vi "s-lab第7章 程序结构1-20.vi"() -> ()   [LabVIEW 2013]
uses:
  <vilib>/Platform/TimedLoop/XDataNode/timing_clust.ctl
  <vilib>/Platform/TimedLoop/XDataNode/nitl_modes.ctl
  <vilib>/Platform/TimedLoop/XDataNode/wakeup.ctl
  <vilib>/Platform/TimedLoop/XDataNode/XDataNode.xnode
  <vilib>/Platform/TimedLoop/XDataNode/XDNodeRunTimeDep.lvlib
panel:
  out "平方根":dbl
  in  "数值 8":dbl
  out "判断结果":dbl
  in  "比较门限":dbl
  out "随机数":dbl
  out "滑动杆值":dbl
  out "布尔 4":bool
  in  "数值 7":dbl
  in  "滑动杆 3":dbl(slide) scale=0.0..10.0
  out "字符串 5":string
  out "0-n的平方和":dbl
  in  "输入n":dbl
  out "0-99之间的所有偶数之和":dbl
  in  "循环值":dbl
  out "小数":dbl
  out "大数":dbl
  out "循环次数":dbl
  out "字符串 4":string
  in  "字符串 3":string
  out "数值 6":dbl
  in  "数值 5":dbl
  in  "确定按钮":bool
  in  "滑动杆 2":dbl(slide) scale=0.0..10.0
  out "OUT":dbl
  in  "IN":dbl
  out "延迟时间 S 2":dbl
  in  "数值 4":dbl
  out "延迟时间 S":dbl
  in  "数值 3":dbl
  out "数值 2":dbl
  out "字符串 2":string
  in  "停止 2":bool
  out "布尔":bool
  in  "数值":dbl
  in  "滑动杆":dbl(slide) scale=0.0..10.0
  in  "布尔 3":bool
  out "字符串":string
  out "布尔 2":bool
  out "n的和 1":dbl
  in  "数值n 2":dbl
  out "循环数2":dbl
  out "n！ 1":dbl
  in  "数值n 1":dbl
  in  "停止":bool
  out "随机数":dbl
  out "循环数":dbl
  out "n的和":dbl
  in  "数值n":dbl
  out "n！":dbl
  in  "n":dbl
  out "随机数":dbl
  out "循环":dbl
  # "例 1"
  # "例 2"
  # "例 3"
  # "例 4"
  # "例 5"
  # "例 6"
  # "例 7"
  # "例 8"
  # "例 9"
  # "例 10"
  # "例 11"
  # "例 12"
  # "例 13"
  # "例 14"
  # "例 15"
  # "例 16"
  # "例 17"
  # "例 18"
  # "例 19"
  # "例 20"
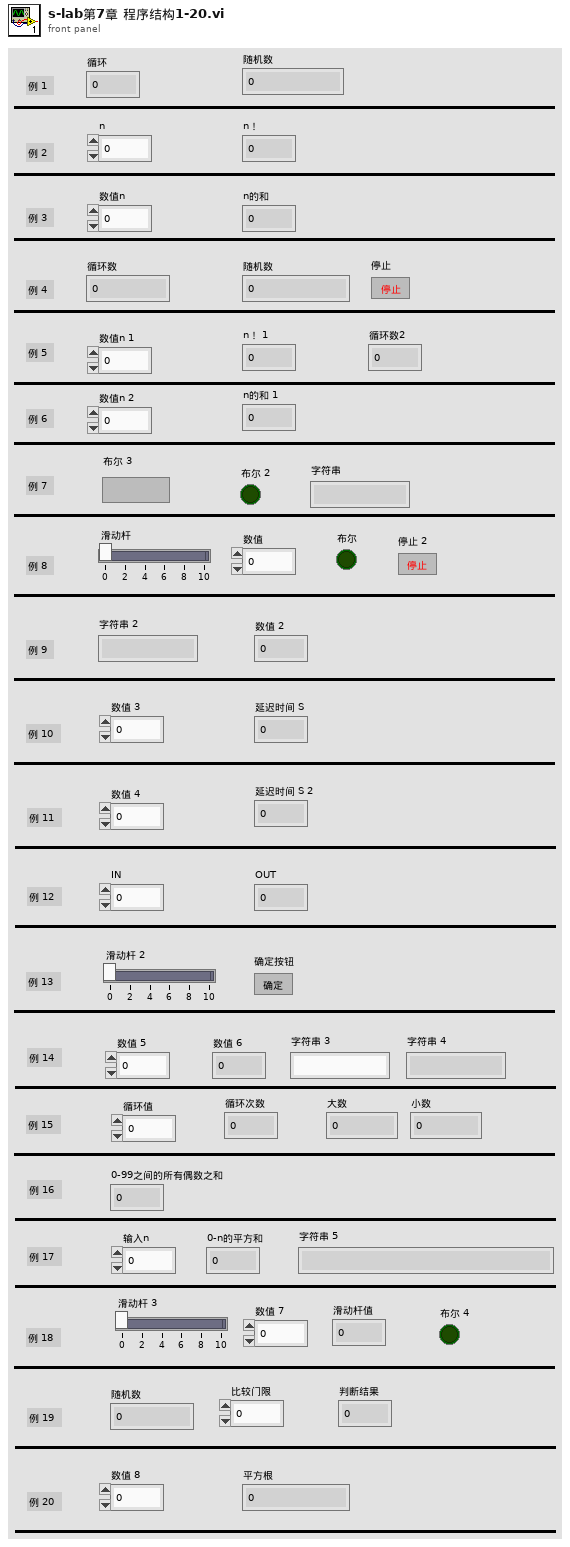
[diagram p1: front panel]
types:
  T1 = typedef "XDNodeRunTimeDep.lvlib/timing_clust.ctl" = cluster{"Expected End [f-1]":u64, "Actual End [f-1]":u64, "Finished Late? [f-1]":bool, "Expected End [i-1]":u64, "Actual End [i-1]":u64, "Finished Late? [i-1]":bool, "Expected Start [i]":u64, "Actual Start [i]":u64, "Expected Start [f]":u64, "Actual Start [f]":u64, "Source Name":string, "Structure Name":string, "Period":i64, "Deadline":i64, "Offset":i64, "Start":i64, "Priority":i32, "Timeout":i32, "Mode":T2, "Wakeup Reason":T3, "Error":errorcluster, "Source Type":string, "Secondary Source Type":string, "Global End Time":u64, "Global Start Time":u64, "Frame Duration":u64, "Iteration Duration":u64, "Assigned CPU":i32, "I/O Scan Engine Mode":u32}
  T2 = typedef "XDNodeRunTimeDep.lvlib/nitl_modes.ctl" = enum32{"No Change", "Process missed periods, maintain original phase", "Discard missed periods, maintain original phase", "Process missed periods, ignore original phase", "Discard missed periods, ignore original phase"}
  T3 = typedef "XDNodeRunTimeDep.lvlib/wakeup.ctl" = enum32{"Normal", "Aborted", "Asynchronous wakeup", "Timing source error", "Timed loop error", "Timeout"}
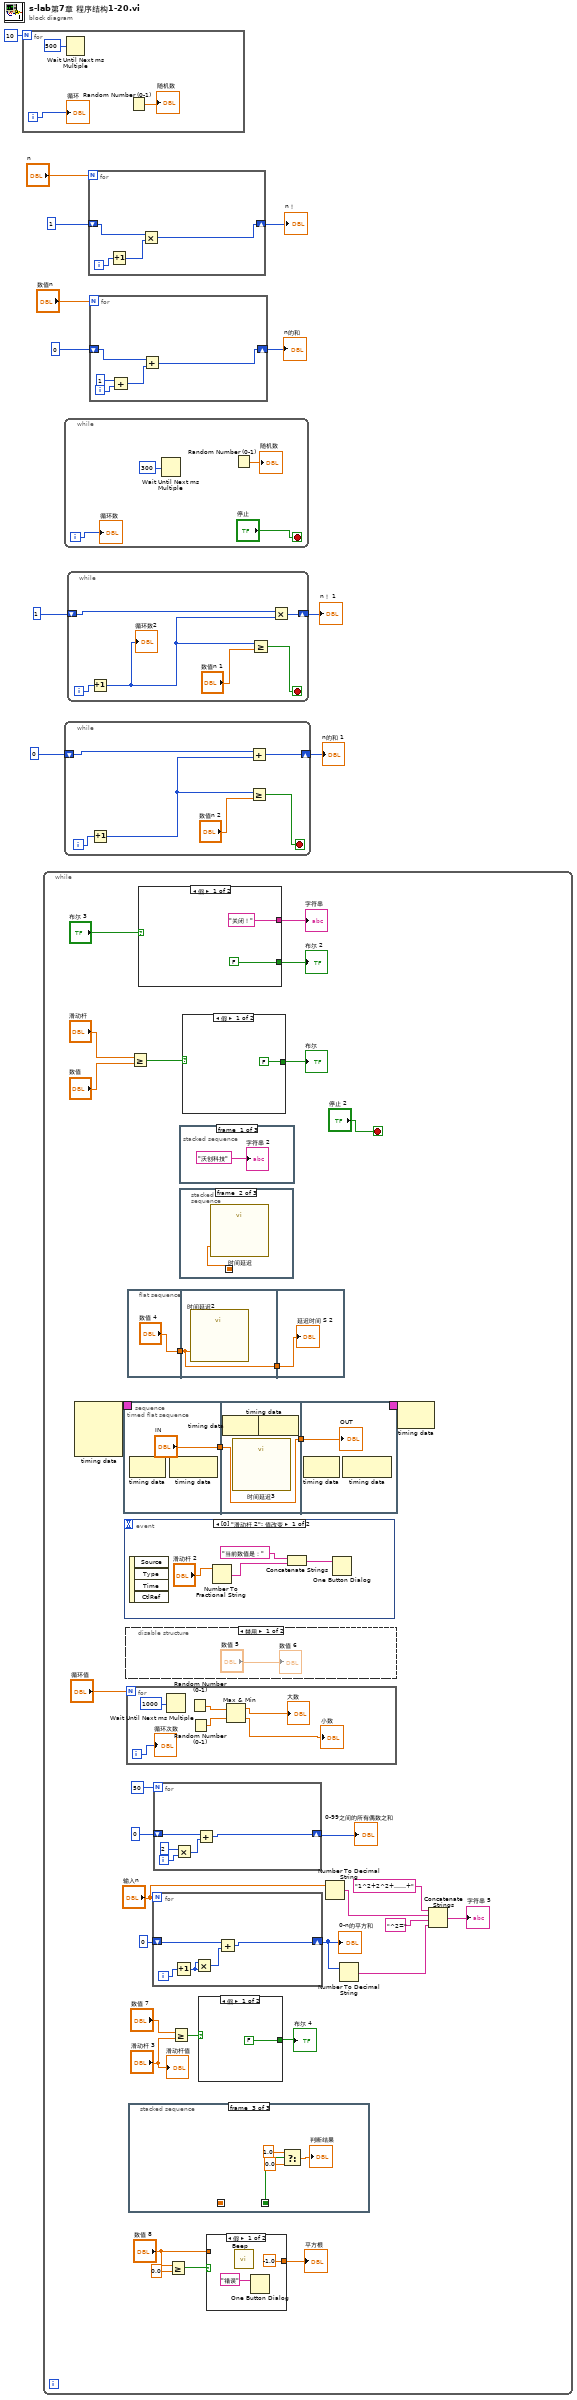
[diagram p0: block diagram]
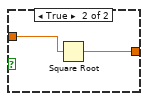
[diagram p2: hidden frame]
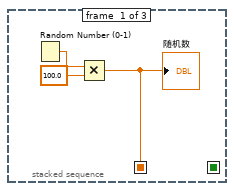
[diagram p3: hidden frame]
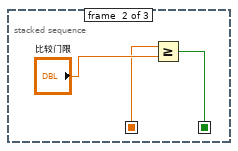
[diagram p4: hidden frame]
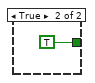
[diagram p5: hidden frame]
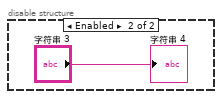
[diagram p6: hidden frame]
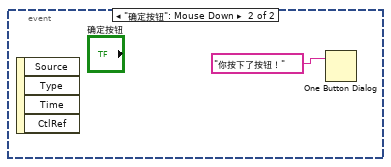
[diagram p7: hidden frame]
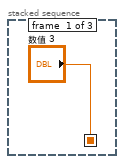
[diagram p8: hidden frame]
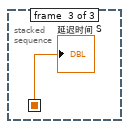
[diagram p9: hidden frame]
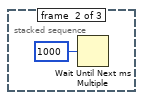
[diagram p10: hidden frame]
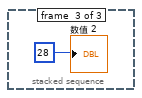
[diagram p11: hidden frame]
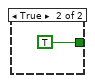
[diagram p12: hidden frame]
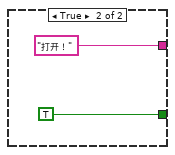
[diagram p13: hidden frame]
diagram:
  n1 = for {
    N: 10 -> [_]
    i -> [w12]
    n2 = Wait Until Next ms Multiple(millisecond multiple=u32 500 ("毫秒倍数")) -> ()  [unwired: 1 out]
    n3 = Random Number (0-1)() -> (number: 0 to 1=→"随机数":dbl)
    "循环" <- w12
  }
  n4 = while {
    stop <- "停止 2" stop-if-true
    n5 = node-c288() -> (w36:T1)  [unwired: 4 in]
    n6 = timed-sequence {
      timing: w36 -> [_]
      timing-out: [_] -> w35
      n7 = timed-flat-sequence {
        tunnel: ["IN"] -> w86
        tunnel: [w91] -> w87
        tunnel: w86 -> [w91]
        tunnel: w87 -> [w94]
        frame #0 {
          n8 = node-c288() -> ()  [unwired: 1 in, 1 out]
          n9 = node-c288() -> ()  [unwired: 1 in, 1 out]
        }
        frame #1 {
          n10 = node-c288() -> ()  [unwired: 1 in, 1 out]
          n11 = call "时间延迟3"() -> ()  [unwired: 11 in, 1 out]
          n12 = node-c288() -> ()  [unwired: 1 in, 1 out]
        }
        frame #2 {
          n13 = node-c288() -> ()  [unwired: 1 in, 1 out]
          n14 = node-c288() -> ()  [unwired: 1 in, 1 out]
          "OUT" <- w94
        }
      }
    }
    n15 = event shown="[0] \"滑动杆 2\": 值改变" {
      selector: _ -> [_ _]
      dyn-events: _ -> [_ _]
      timeout: _ -> [_ _]
      event "滑动杆 2": Value Change {
        n16 = event-data() -> ()  [unwired: 1 in, 4 out]
        n17 = Number To Fractional String(number="滑动杆 2") -> (F-format string=w83:string)  [unwired: 3 in]
        n18 = Concatenate Strings("当前数值是：", w83) -> (w81:string)
        n19 = One Button Dialog(message=w81) -> ()  [unwired: 1 in, 1 out]
      }
      event "确定按钮": Mouse Down {
        n20 = event-data() -> ()  [unwired: 1 in, 4 out]
        n21 = One Button Dialog(message="你按下了按钮！") -> ()  [unwired: 1 in, 1 out]
      }
    }
    n22 = disable-structure shown="禁用" {
      frame Disabled {
        "数值 6" <- "数值 5"
      }
      frame Enabled {
        "字符串 4" <- "字符串 3"
      }
    }
    n23 = for {
      N: "循环值" -> [_]
      i -> [w78]
      n24 = Wait Until Next ms Multiple(millisecond multiple=u32 1000 ("毫秒倍数")) -> ()  [unwired: 1 out]
      n25 = Random Number (0-1)() -> (number: 0 to 1=w77:dbl)
      n26 = Random Number (0-1)() -> (number: 0 to 1=w76:dbl)
      n27 = Max & Min(x=w77, y=w76) -> (max(x,y)=→"大数":dbl, min(x,y)=→"小数":dbl)
      "循环次数" <- w78
    }
    n28 = flat-sequence {
      tunnel: ["数值 4"] -> w38
      tunnel: w38 -> [w100]
      tunnel: [w100] -> w37
      tunnel: w37 -> [w101]
      frame #0 {
      }
      frame #1 {
        n29 = call "时间延迟2"("Delay Time (s)"=w100) -> ()  [unwired: 10 in, 1 out]
      }
      frame #2 {
        "延迟时间 S 2" <- w101
      }
    }
    n30 = stacked-sequence {
      seq-local: [w51 _ _] -> [_ w55 _]
      seq-local: [_ w54 _] -> [_ _ w59]
      frame #0 {
        n31 = Random Number (0-1)() -> (number: 0 to 1=w53:dbl)
        n32 = Multiply(x=w53, y=100.0) -> (x*y=w51:dbl)
        "随机数" <- w51
      }
      frame #1 {
        n33 = Greater Or Equal?(x=w55, y="比较门限") -> (x >= y?=w54:bool)
      }
      frame #2 {
        n34 = Select(t=1.0, s=w59, f=0.0) -> (s? t:f=→"判断结果":dbl)
      }
    }
    n35 = Greater Or Equal?(x="滑动杆", y="数值") -> (x >= y?=w43:bool)
    n36 = case shown="假" "布尔 3" {
      tunnel: [FALSE TRUE] -> w40
      tunnel: ["关闭！" "打开！"] -> w41
      frame False {
      }
      frame True {
      }
    }
    "布尔 2" <- w40
    "字符串" <- w41
    n37 = for {
      N: "输入n" -> [_]
      shift-right: [w63] -> w29
      shift-left: 0 -> [w64]
      i -> [w67]
      n38 = Increment(x=w67) -> (x+1=w66:i32)
      n39 = Multiply(x=w66, y=w66) -> (x*y=w65:i32)
      n40 = Add(x=w64, y=w65) -> (x+y=w63:i32)
    }
    "0-n的平方和" <- w29
    n41 = for {
      N: 50 -> [_]
      shift-right: [w68] -> w31
      shift-left: 0 -> [w69]
      i -> [w72]
      n42 = Multiply(x=2, y=w72) -> (x*y=w70:i32)
      n43 = Add(x=w69, y=w70) -> (x+y=w68:i32)
    }
    "0-99之间的所有偶数之和" <- w31
    n44 = Greater Or Equal?(x="数值 8", y=0.0) -> (x >= y?=w17:bool)
    n45 = Greater Or Equal?(x="数值 7", y="滑动杆 3") -> (x >= y?=w20:bool)
    n46 = stacked-sequence {
      seq-local: ["数值 3" _ _] -> [_ w103 w104]
      frame #0 {
      }
      frame #1 {
        n47 = call "时间延迟"("Delay Time (s)"=w103) -> ()  [unwired: 10 in, 1 out]
      }
      frame #2 {
        "延迟时间 S" <- w104
      }
    }
    n48 = stacked-sequence {
      frame #0 {
        "字符串 2" <- "沃创科技"
      }
      frame #1 {
        n49 = Wait Until Next ms Multiple(millisecond multiple=u32 1000 ("毫秒倍数")) -> ()  [unwired: 1 out]
      }
      frame #2 {
        "数值 2" <- 28
      }
    }
    n50 = case shown="假" w43 {
      tunnel: [FALSE TRUE] -> w46
      frame False {
      }
      frame True {
      }
    }
    "布尔" <- w46
    n51 = case shown="假" w20 {
      tunnel: [FALSE TRUE] -> w19
      frame False {
      }
      frame True {
      }
    }
    "布尔 4" <- w19
    n52 = case shown="假" w17 {
      tunnel: "数值 8" -> [_ w50]
      tunnel: [-1.0 w49] -> w15
      frame False {
        n53 = call <vilib>:"Beep.vi"() -> ()  [unwired: 12 in]
        n54 = One Button Dialog(message="错误") -> ()  [unwired: 1 in, 1 out]
      }
      frame True {
        n55 = Square Root(x=w50) -> (sqrt(x)=w49:dbl)
      }
    }
    "平方根" <- w15
    n56 = Number To Decimal String(number="输入n") -> (decimal integer string=w25:string)  [unwired: 1 in]
    n57 = Number To Decimal String(number=w29) -> (decimal integer string=w27:string)  [unwired: 1 in]
    n58 = node-c288(w35) -> ()  [unwired: 1 out]
    n59 = Concatenate Strings("1^2+2^2+……+", w25, "^2=", w27) -> (→"字符串 5":string)
    "滑动杆值" <- "滑动杆 3"
  }
  n60 = while {
    i -> [w116]
    stop <- "停止" stop-if-true
    n61 = Wait Until Next ms Multiple(millisecond multiple=u32 300 ("毫秒倍数")) -> ()  [unwired: 1 out]
    n62 = Random Number (0-1)() -> (number: 0 to 1=→"随机数":dbl)
    "循环数" <- w116
  }
  n63 = while {
    shift-right: [w122] -> w1
    shift-left: 0 -> [w121]
    i -> [w123]
    stop <- w120 stop-if-true
    n64 = Increment(x=w123) -> (x+1=w118:i32)
    n65 = Add(x=w121, y=w118) -> (x+y=w122:i32)
    n66 = Greater Or Equal?(x=w118, y="数值n 2") -> (x >= y?=w120:bool)
  }
  "n的和 1" <- w1
  n67 = while {
    shift-right: [w128] -> w3
    shift-left: 1 -> [w127]
    i -> [w129]
    stop <- w126 stop-if-true
    n68 = Increment(x=w129) -> (x+1=w124:i32)
    "循环数2" <- w124
    n69 = Greater Or Equal?(x=w124, y="数值n 1") -> (x >= y?=w126:bool)
    n70 = Multiply(x=w127, y=w124) -> (x*y=w128:i32)
  }
  "n！ 1" <- w3
  n71 = for {
    N: "n" -> [_]
    shift-right: [w131] -> w8
    shift-left: 1 -> [w132]
    i -> [w130]
    n72 = Increment(x=w130) -> (x+1=w133:i32)
    n73 = Multiply(x=w132, y=w133) -> (x*y=w131:i32)
  }
  "n！" <- w8
  n74 = for {
    N: "数值n" -> [_]
    shift-right: [w134] -> w6
    shift-left: 0 -> [w135]
    i -> [w138]
    n75 = Add(x=1, y=w138) -> (x+y=w136:i32)
    n76 = Add(x=w135, y=w136) -> (x+y=w134:i32)
  }
  "n的和" <- w6
